vi "GetTagsByProperty.vi"(10 "property":T1, 11 "tags":T2[](array[typedef])) -> (3 "matches":T2[](array[typedef]))   [LabVIEW 2017, in "DeviceModelHelpers.lvlib"]
uses:
  <vilib>/addons/InsightCM/Utilities/DeviceModelHelpers/DeviceModelHelpers.lvlib
  <vilib>/addons/InsightCM/MessageBus/Base/controls/Tag.ctl
  <vilib>/addons/InsightCM/MessageBus/Base/controls/KeyValuePair.ctl
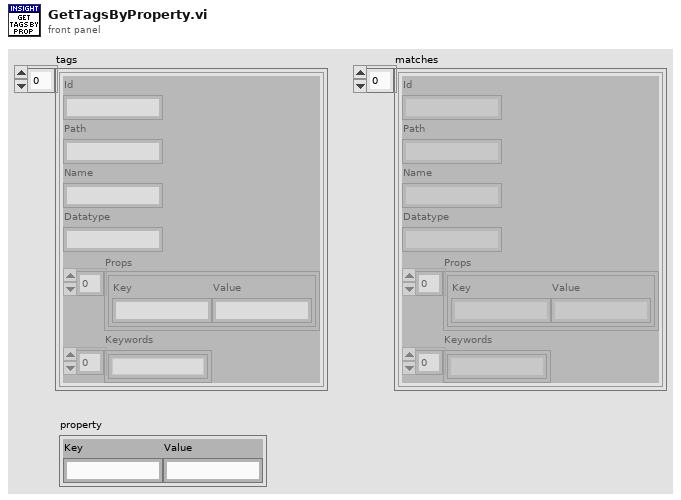
[diagram p1: front panel]
types:
  T1 = typedef "KeyValuePair.ctl" = cluster{"Key":string, "Value":string}
  T2 = typedef "Tag.ctl" = cluster{"Id":string, "Path":string, "Name":string, "Datatype":string, "Props":T1[], "Keywords":string[]}
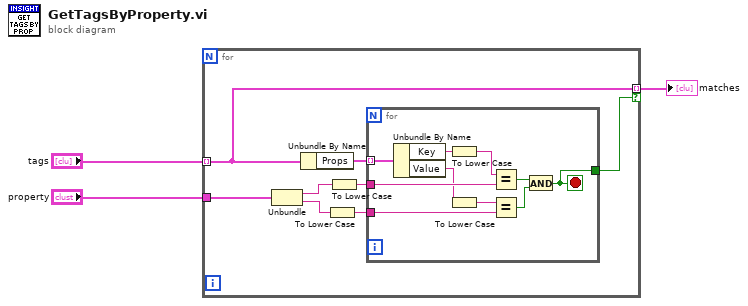
[diagram p0: block diagram]
diagram:
  n1 = for {
    tunnel: "tags" -> [w5] mode=indexing
    tunnel: "property" -> [w11]
    tunnel: [w5] -> w1 mode=indexing if=w4
    n2 = Unbundle(w11) -> ("Key"=w7:string, "Value"=w6:string)
    n3 = Unbundle By Name(w5) -> ("Props"=w10:T1[])
    n4 = To Lower Case(string=w6) -> (all lower case string=w9:string)
    n5 = To Lower Case(string=w7) -> (all lower case string=w8:string)
    n6 = for {
      tunnel: w8 -> [w21]
      tunnel: [w14] -> w4
      tunnel: w10 -> [w20] mode=indexing
      tunnel: w9 -> [w16]
      stop <- w14 stop-if-true
      n7 = Unbundle By Name(w20) -> ("Key"=w18:string, "Value"=w17:string)
      n8 = To Lower Case(string=w18) -> (all lower case string=w13:string)
      n9 = To Lower Case(string=w17) -> (all lower case string=w12:string)
      n10 = Equal?(x=w13, y=w21) -> (x = y?=w19:bool)
      n11 = Equal?(x=w12, y=w16) -> (x = y?=w15:bool)
      n12 = And(x=w19, y=w15) -> (x .and. y?=w14:bool)
    }
  }
  "matches" <- w1
